vi "T1_viewer_gui_exe.vi"() -> ()   [LabVIEW 2014]
panel:
  out "progress":u8(slide) scale=0.0..100.0
  in  "normalize":bool
  out "t1_curves":T1(graph)
  in  "plot":bool
  in  "file_list":i32[](listbox)
  in  "files_folder":path=path "D:/Data/raw data"
  in  "stop":bool
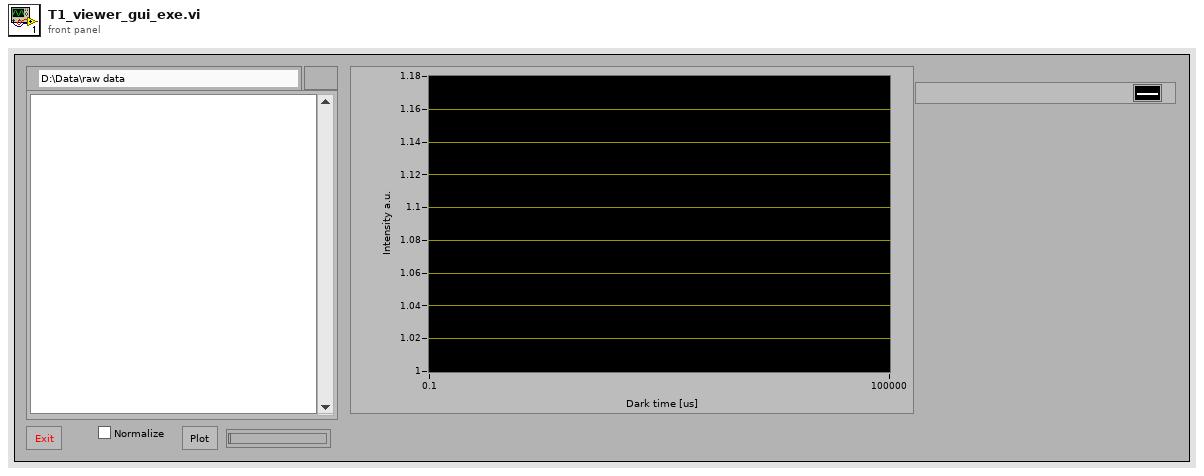
[diagram p1: front panel]
types:
  T1 = cluster{"dark_times_us":dbl[], "measured_signal":dbl[]}[]
  T2 = cluster{"dark_times_us":dbl[], "measured_signal":dbl[]}
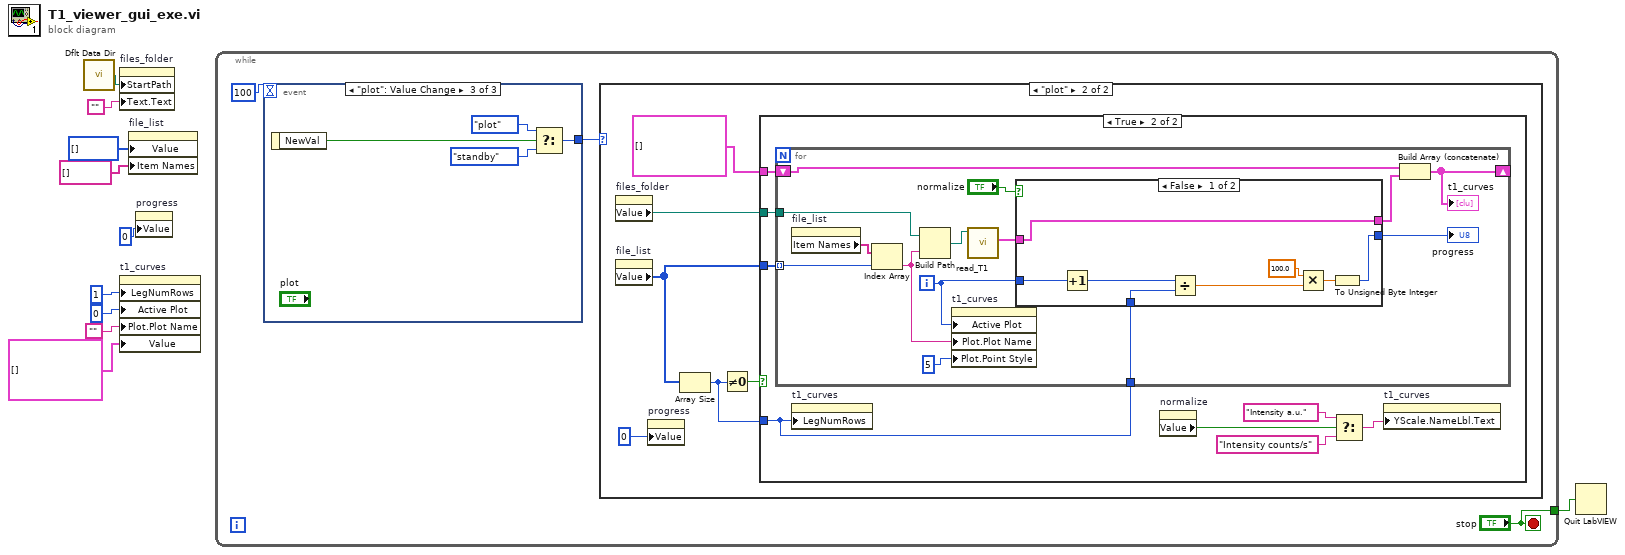
[diagram p0: block diagram]
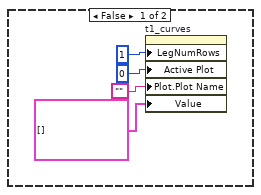
[diagram p3: hidden frame]
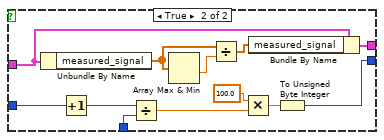
[diagram p4: hidden frame]
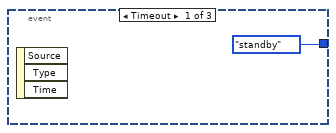
[diagram p5: hidden frame]
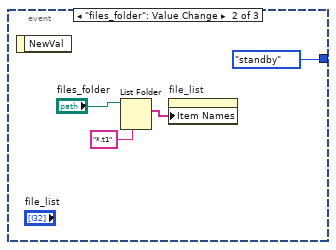
[diagram p6: hidden frame]
diagram:
  n1 = call <vilib>:"Dflt Data Dir.vi"() -> ("App:Default Data Directory"=w8:path)
  n2 = property on="files_folder" class="Path"("StartPath"=w8, "Text.Text"="") -> ()  [unwired: 2 in, 2 out]
  n3 = property on="t1_curves" class="XYGraph (strict)"("LegNumRows"=u32 1 ("Legend:Number of Rows"), "Active Plot"=u32 0, "Plot.Plot Name"="", "Value"=T1 [] ("t1_curves")) -> ()  [unwired: 2 in, 2 out]
  n4 = property on="file_list" class="LstBox (strict)"("Value"=i32[] [] ("file_list"), "Item Names"=string[] []) -> ()  [unwired: 2 in, 2 out]
  n5 = property on="progress" class="Slide (strict)"("Value"=u8 0 ("progress")) -> ()  [unwired: 2 in, 2 out]
  n6 = while {
    tunnel: ["stop"] -> w1
    stop <- "stop" stop-if-true
    n7 = event shown="[2] \"plot\": Value Change" {
      selector: _ -> [_ _ _]
      dyn-events: _ -> [_ _ _]
      timeout: 100 -> [_ _ _]
      tunnel: [enum16{"standby", "plot"}."standby" enum16{"standby", "plot"}."standby" w71] -> w12
      event Timeout {
        n8 = event-data() -> ()  [unwired: 1 in, 3 out]
      }
      event "files_folder": Value Change {
        n9 = event-data() -> ()  [unwired: 1 in, 1 out]
        n10 = List Folder(path="files_folder", pattern="*.t1") -> (filenames=w68:string[])  [unwired: 2 in, 3 out]
        n11 = property on="file_list" class="LstBox (strict)"("Item Names"=w68) -> ()  [unwired: 2 in, 2 out]
      }
      event "plot": Value Change {
        n12 = event-data() -> ("NewVal"=w72:bool)  [unwired: 1 in]
        n13 = Select(t=enum16{"standby", "plot"}."plot", s=w72, f=enum16{"standby", "plot"}."standby") -> (s? t:f=w71:enum16{"standby", "plot"})
      }
    }
    n14 = case shown="\"plot\"" w12 {
      frame "standby", Default {
      }
      frame "plot" {
        n15 = property on="files_folder" class="Path"() -> ("Value"=w19:path)  [unwired: 2 in, 2 out]
        n16 = property on="file_list" class="LstBox (strict)"() -> ("Value"=w18:i32[])  [unwired: 2 in, 2 out]
        n17 = property on="progress" class="Slide (strict)"("Value"=u8 0 ("progress")) -> ()  [unwired: 2 in, 2 out]
        n18 = Array Size(array=w18) -> (size(s)=w16:i32)
        n19 = Not Equal To 0?(x=w16) -> (x != 0?=w17:bool)
        n20 = case shown="True" w17 {
          tunnel: w19 -> [_ w31]
          tunnel: w18 -> [_ w30]
          tunnel: w16 -> [_ w29]
          tunnel: T1 [] ("t1_curves") -> [_ w28]
          frame False {
            n21 = property on="t1_curves" class="XYGraph (strict)"("LegNumRows"=u32 1 ("Legend:Number of Rows"), "Active Plot"=u32 0, "Plot.Plot Name"="", "Value"=T1 [] ("t1_curves")) -> ()  [unwired: 2 in, 2 out]
          }
          frame True {
            n22 = for {
              tunnel: w30 -> [w45] mode=indexing
              tunnel: w31 -> [w42]
              tunnel: w29 -> [w36]
              shift-right: [w33] -> _
              shift-left: w28 -> [w34]
              i -> [w37]
              n23 = property on="file_list" class="LstBox (strict)"() -> ("Item Names"=w44:string[])  [unwired: 2 in, 2 out]
              n24 = Index Array(array=w44, index=w45) -> (element=w38:string)
              n25 = Build Path(base path=w42, name or relative path=w38) -> (appended path=w43:path)
              n26 = property on="t1_curves" class="XYGraph (strict)"("Active Plot"=w37, "Plot.Plot Name"=w38, "Plot.Point Style"=u8 5) -> ()  [unwired: 2 in, 2 out]
              n27 = call "read_T1.vi"("file_path"=w43) -> ("T1_curve"=w41:T2)  [unwired: 4 in, 6 out]
              n28 = case shown="False" "normalize" {
                tunnel: w41 -> [w53 w64]
                tunnel: [w53 w62] -> w35
                tunnel: w37 -> [w52 w59]
                tunnel: w36 -> [w51 w60]
                tunnel: [w47 w54] -> w32
                frame False {
                  n29 = Increment(x=w52) -> (x+1=w46:i32)
                  n30 = Divide(x=w46, y=w51) -> (x/y=w48:dbl)
                  n31 = Multiply(x=100.0, y=w48) -> (x*y=w49:dbl)
                  n32 = To Unsigned Byte Integer(number=w49) -> (unsigned 8bit integer=w47:u8)
                }
                frame True {
                  n33 = Unbundle By Name(w64) -> ("measured_signal"=w65:dbl[])
                  n34 = Increment(x=w59) -> (x+1=w58:i32)
                  n35 = Divide(x=w58, y=w60) -> (x/y=w56:dbl)
                  n36 = Array Max & Min(array=w65) -> (min value=w61:dbl)  [unwired: 3 out]
                  n37 = Divide(x=w65, y=w61) -> (x/y=w63:dbl[])
                  n38 = Multiply(x=100.0, y=w56) -> (x*y=w55:dbl)
                  n39 = Bundle By Name(cluster=w64, "measured_signal"=w63) -> (w62:T2)
                  n40 = To Unsigned Byte Integer(number=w55) -> (unsigned 8bit integer=w54:u8)
                }
              }
              "progress" <- w32
              n41 = Build Array (concatenate)(w34, w35) -> (w33:T1)
              "t1_curves" <- w33
            }
            n42 = property on="t1_curves" class="XYGraph (strict)"("LegNumRows"=w29) -> ()  [unwired: 2 in, 2 out]
            n43 = property on="normalize" class="Bool (strict)"() -> ("Value"=w27:bool)  [unwired: 2 in, 2 out]
            n44 = Select(t="Intensity a.u.", s=w27, f="Intensity counts/s") -> (s? t:f=w26:string)
            n45 = property on="t1_curves" class="XYGraph (strict)"("YScale.NameLbl.Text"=w26) -> ()  [unwired: 2 in, 2 out]
          }
        }
      }
    }
  }
  n46 = Quit LabVIEW(quit? (T)=w1) -> ()
